vi "Set Pixel Mode.vi"(10 "colormode":i32, 11 "bitdepth":i32) -> (3 "function return":u32)   [LabVIEW 2018, in "AndorSDK.lvlib"]
doc: "EXPNETTYPE unsigned int WINAPI SetPixelMode(int bitdepth, int colormode);"
uses:
  AndorSDK.lvlib
  ATMCD32D.dll
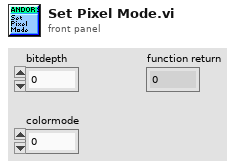
[diagram p1: front panel]
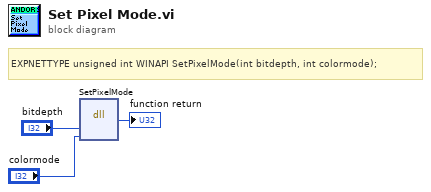
[diagram p0: block diagram]
diagram:
  # "EXPNETTYPE unsigned int WINAPI SetPixelMode(int bitdepth, int colormode);"
  n1 = dll-call lib="PTH2babs E\nPersönliches02 - Arbeit03-HiwijobsLabviewCodelibANDOR\tAndor SDK\nATMCD32D.*" fn="SetPixelMode"("bitdepth"="bitdepth", "colormode"="colormode") -> (→"function return":u32)  [unwired: 5 in, 2 out]
